vi "GolecMelody (SubVI).vi"() -> (3 "Melody (Frequency:Duration)":i32[][](array[numeric])=[[466, 1], [933, 1], [232, 1], [261, 250], [261, 125], [232, 125], [261, 125], [329, 125], [391, 125], [440, 1000], [349, 250], [523, 250], [391, 63], [349, 63], [391, 500], [391, 1000], [261, 250], [261, 125], [194, 125], [261, 125], [329, 125], [391, 125], [466, 1], [933, 1], [232, 1], [440, 500], [466, 250], [440, 125], [466, 250], [391, 63], [349, 63], [0, 250], [329, 63], [349, 63], [391, 500], [391, 1000], [194, 125], [219, 125], [0, 250], [219, 125], [232, 125], [0, 250], [232, 125], [261, 125], [466, 1], [294, 125], [0, 250], [294, 125], [466, 1], [933, 1], [232, 1], [329, 125], [0, 250], [329, 125], [349, 125], [466, 1], [391, 125], [0, 250], [391, 125], [0, 125], [0, 250], [261, 125], [466, 1], [329, 250], [294, 125], [261, 250], [261, 250], [261, 250], [232, 125], [219, 1250], [0, 250], [194, 125], [232, 125], [0, 250], [0, 125], [232, 250], [219, 125], [466, 1], [933, 1], [232, 1], [194, 250], [0, 250], [5, 500], [261, 250], [329, 125], [294, 125], [294, 125], [261, 125], [0, 125], [261, 125], [261, 250], [261, 250], [232, 125], [219, 125], [0, 250], [194, 250], [232, 250], [0, 250], [232, 125], [219, 125], [194, 250], [0, 250], [0, 500], [261, 250], [329, 125], [294, 125], [261, 125], [0, 250], [261, 250], [261, 125], [232, 125], [219, 125], [0, 250], [194, 125], [232, 125], [0, 250], [0, 125], [232, 250], [219, 125], [194, 500], [0, 500], [0, 125], [329, 250], [329, 125], [294, 125], [261, 125], [0, 250], [261, 125], [261, 250], [232, 125], [219, 125], [0, 250], [194, 250], [232, 125], [0, 125], [0, 125], [232, 250], [219, 125], [194, 500], [0, 500], [261, 375], [194, 375], [261, 125], [194, 125], [261, 125], [219, 125], [261, 188], [219, 188], [294, 375], [232, 375], [294, 125], [232, 125], [0, 250], [294, 125], [232, 125], [294, 125], [232, 125], [0, 250], [329, 375], [261, 375], [329, 125], [261, 125], [349, 125], [294, 125], [232, 375], [466, 250], [391, 250], [440, 250], [349, 250], [391, 250], [329, 250], [349, 250], [294, 250], [0, 125], [0, 125], [261, 250], [194, 250], [294, 125], [329, 125], [261, 125], [391, 375], [370, 375], [311, 375], [415, 125], [370, 125], [311, 125], [415, 125], [0, 250], [415, 125], [311, 125], [370, 375], [329, 125], [232, 125], [294, 375], [261, 125], [185, 250], [207, 125], [329, 125], [311, 250], [232, 188]])   [LabVIEW 2014]
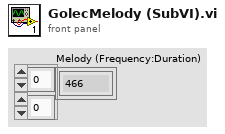
[diagram p1: front panel]
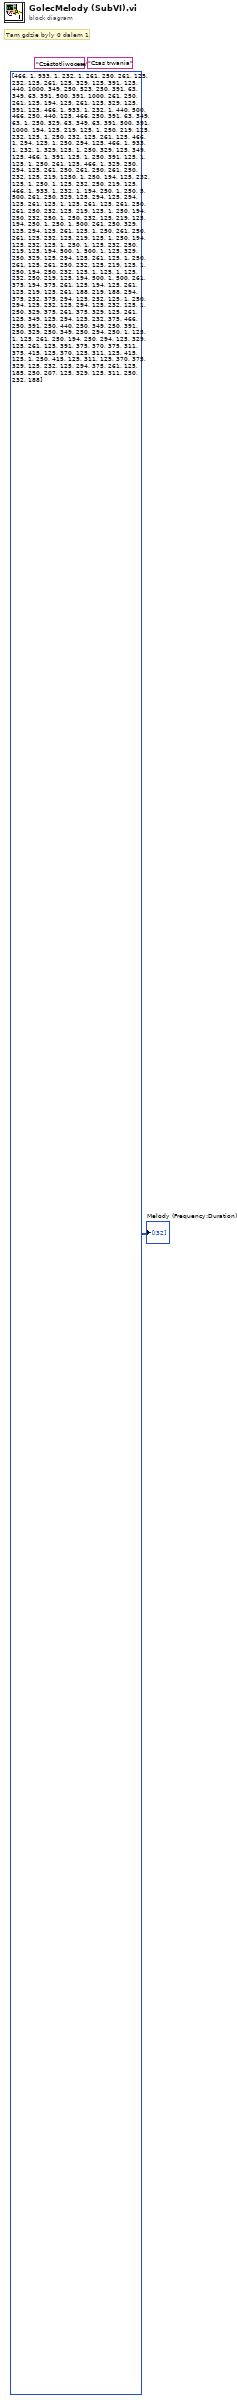
[diagram p0: block diagram]
diagram:
  (unwired) "Czas trwania"
  (unwired) "Czêstotliwoœæ"
  # "Tam gdzie byly 0 dalem 1"
  "Melody (Frequency:Duration)" <- i32[][] [[466, 1], [933, 1], [232, 1], [261, 250], [261, 125], [232, 125], [261, 125], [329, 125], [391, 125], [440, 1000], [349, 250], [523, 250], [391, 63], [349, 63], [391, 500], [391, 1000], [261, 250], [261, 125], [194, 125], [261, 125], [329, 125], [391, 125], [466, 1], [933, 1], [232, 1], [440, 500], [466, 250], [440, 125], [466, 250], [391, 63], [349, 63], [1, 250], [329, 63], [349, 63], [391, 500], [391, 1000], [194, 125], [219, 125], [1, 250], [219, 125], [232, 125], [1, 250], [232, 125], [261, 125], [466, 1], [294, 125], [1, 250], [294, 125], [466, 1], [933, 1], [232, 1], [329, 125], [1, 250], [329, 125], [349, 125], [466, 1], [391, 125], [1, 250], [391, 125], [1, 125], [1, 250], [261, 125], [466, 1], [329, 250], [294, 125], [261, 250], [261, 250], [261, 250], [232, 125], [219, 1250], [1, 250], [194, 125], [232, 125], [1, 250], [1, 125], [232, 250], [219, 125], [466, 1], [933, 1], [232, 1], [194, 250], [1, 250], [5, 500], [261, 250], [329, 125], [294, 125], [294, 125], [261, 125], [1, 125], [261, 125], [261, 250], [261, 250], [232, 125], [219, 125], [1, 250], [194, 250], [232, 250], [1, 250], [232, 125], [219, 125], [194, 250], [1, 250], [1, 500], [261, 250], [329, 125], [294, 125], [261, 125], [1, 250], [261, 250], [261, 125], [232, 125], [219, 125], [1, 250], [194, 125], [232, 125], [1, 250], [1, 125], [232, 250], [219, 125], [194, 500], [1, 500], [1, 125], [329, 250], [329, 125], [294, 125], [261, 125], [1, 250], [261, 125], [261, 250], [232, 125], [219, 125], [1, 250], [194, 250], [232, 125], [1, 125], [1, 125], [232, 250], [219, 125], [194, 500], [1, 500], [261, 375], [194, 375], [261, 125], [194, 125], [261, 125], [219, 125], [261, 188], [219, 188], [294, 375], [232, 375], [294, 125], [232, 125], [1, 250], [294, 125], [232, 125], [294, 125], [232, 125], [1, 250], [329, 375], [261, 375], [329, 125], [261, 125], [349, 125], [294, 125], [232, 375], [466, 250], [391, 250], [440, 250], [349, 250], [391, 250], [329, 250], [349, 250], [294, 250], [1, 125], [1, 125], [261, 250], [194, 250], [294, 125], [329, 125], [261, 125], [391, 375], [370, 375], [311, 375], [415, 125], [370, 125], [311, 125], [415, 125], [1, 250], [415, 125], [311, 125], [370, 375], [329, 125], [232, 125], [294, 375], [261, 125], [185, 250], [207, 125], [329, 125], [311, 250], [232, 188]]
